vi "Test Window Position.vi"(11 "Test Case In":refnum<class "Editor Position.lvclass">) -> (0 "error out":errorcluster, 3 "Test Case Out":refnum<class "Editor Position.lvclass">)   [LabVIEW 2021, in "Editor Position.lvclass"]
uses:
  Editor Position.lvclass
  <vilib>/Astemes/LUnit/Test Case.lvclass/Test Case.ctl
  Editor Position.lvclass/Editor Position.ctl
  4993e8ee-a06a-463a-9684-69129f64d5ce.vi
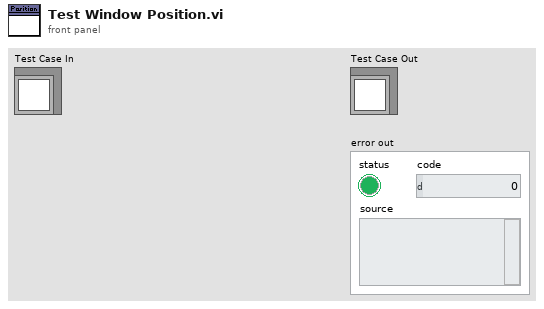
[diagram p1: front panel]
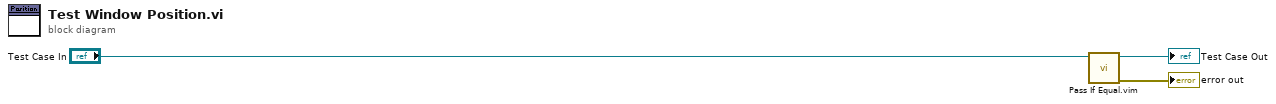
[diagram p0: block diagram]
diagram:
  n1 = call "Pass If Equal.vim"("LUnit Test Case In"="Test Case In") -> ("error out"=→"error out":errorcluster, "LUnit Test Case Out"=→"Test Case Out":refnum<class "Editor Position.lvclass">)  [unwired: 9 in]
